vi "Write All Elements Hidden.vi"(8 "error in (no error)":errorcluster, 10 "Acquis. params. hidden":T1={"Image acquisition timeout factor"=1.0, "Image collection timeout factor"=2.0, "Manual trigger ID"=25, "Precision hardware counter"="Dev1/ctr0", "When to use gate signal?"=FALSE, "Minimum acquisition timeout"=0, "External timing channel"="/Dev1/PFI4", "External gating channel"=""}, 11 "Acquis params in":refnum<class "CV-Acquisition.lvclass">) -> (0 "error out":errorcluster, 3 "Acquis params out":refnum<class "CV-Acquisition.lvclass">)   [LabVIEW 2013, in "CameraVision.lvlib" / "CV-Acquisition.lvclass"]
uses:
  CV-Acquisition.lvclass
  Acquisition-parameters-advanced.ctl
  CV-Acquisition.lvclass/CV-Acquisition.ctl
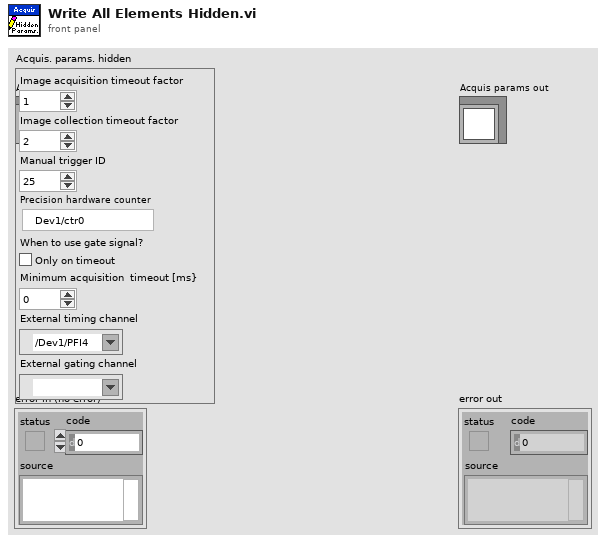
[diagram p1: front panel]
types:
  T1 = typedef "CameraVision.lvlib/CV-Acquisition.lvclass/Acquisition-parameters-advanced.ctl" = cluster{"Image acquisition timeout factor":dbl, "Image collection timeout factor":dbl, "Manual trigger ID":u8, "Precision hardware counter":tag, "When to use gate signal?":bool, "Minimum acquisition timeout":i32, "External timing channel":tag, "External gating channel":tag}
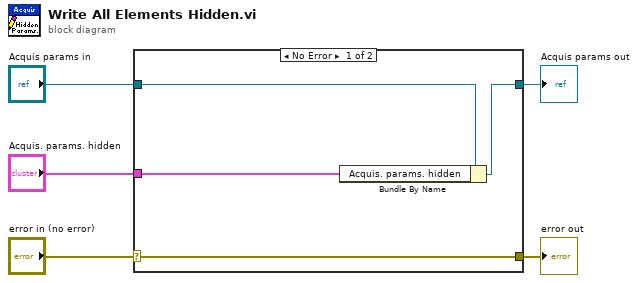
[diagram p0: block diagram]
diagram:
  n1 = case shown="No Error" "error in (no error)" {
    selector: "error in (no error)" -> [w9 w10]
    tunnel: [w9 w10] -> w4
    tunnel: [w7 w11] -> w2
    tunnel: "Acquis params in" -> [w8 w11]
    tunnel: "Acquis. params. hidden" -> [w6 _]
    frame No Error {
      n2 = Bundle By Name(cluster=w8, "Acquis. params. hidden"=w6) -> (w7:refnum<class "CV-Acquisition.lvclass">)
    }
    frame Error {
    }
  }
  "error out" <- w4
  "Acquis params out" <- w2
